vi "Configure Control Mode.vi"(0 "VISA resource name":refnum<visa-resource-name>, 1 "Power Up Enable (F: Off)":bool, 5 "Loop (1:Loop 1)":u16(ring)=1 items=["Loop 1"=1, "Loop 2"=2], 7 "Mode (1:Manual PID)":u16(ring)=1 items=["Manual PID"=1, "Zone"=2, "Open Loop"=3, "AutoTune PID"=4, "AutoTune PI"=5, "AutoTune P"=6], 9 "Control Input (0:A)":u16(ring) items=["A", "B"], 11 "error in (no error)":errorcluster, 12 "Setpoint Units (1:Kelvin)":u16(ring)=1 items=["Kelvin"=1, "Celsius"=2, "Sensor Units"=3], 13 "Heater Output Display (1:Current)":u16(ring)=1 items=["Current"=1, "Power"=2]) -> (4 "VISA resource name out":refnum<visa-resource-name>, 15 "error out":errorcluster)   [LabVIEW 2019, in "Lake Shore 325.lvlib"]
doc: "This VI Specifies the control mode and control loop parameters for the selected loop. The Model 325 has two control modes, Closed Loop and Open Loop. During closed loop control operation the Control Input, Setpoint, Heater Range, PID, and Manual Heater Power (MHP) output parameters are active. Open loop control mode allows the user to directly set the heater output for Loop 1, control output for Loop 2 with the MHP Output parameter.\n\nLoop parameters configured are Input, Setpoint Units, Powerup Enable, and heater output display mode."
uses:
  Lake Shore 325.lvlib
  Instance           2 30Saved   Configure Control Mode .vi
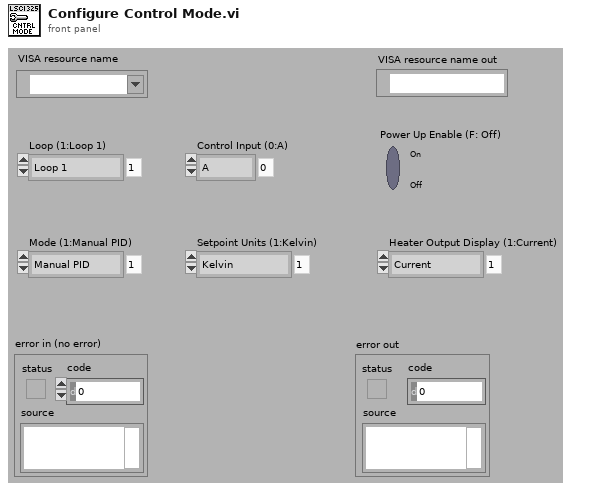
[diagram p1: front panel]
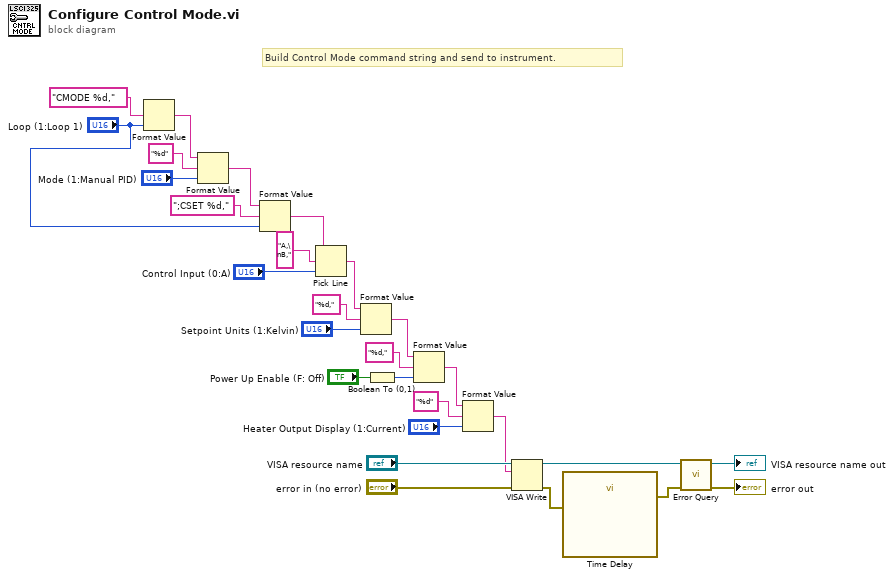
[diagram p0: block diagram]
diagram:
  # "Build Control Mode command string and send to instrument."
  n1 = Format Value(format string="CMODE %d,", value (0)="Loop (1:Loop 1)") -> (output string=w23:string)  [unwired: 1 in]
  n2 = Format Value(string ("")=w23, format string="%d", value (0)="Mode (1:Manual PID)") -> (output string=w18:string)
  n3 = Format Value(string ("")=w18, format string=";CSET %d,", value (0)="Loop (1:Loop 1)") -> (output string=w5:string)
  n4 = Pick Line(string ("")=w5, multi-line string="A,\nB,", line index="Control Input (0:A)") -> (output string=w4:string)
  n5 = Format Value(string ("")=w4, format string="%d,", value (0)="Setpoint Units (1:Kelvin)") -> (output string=w13:string)
  n6 = Boolean To (0,1)(Boolean="Power Up Enable (F: Off)") -> (0, 1=w12:i16)
  n7 = Format Value(string ("")=w13, format string="%d,", value (0)=w12) -> (output string=w9:string)
  n8 = Format Value(string ("")=w9, format string="%d", value (0)="Heater Output Display (1:Current)") -> (output string=w7:string)
  n9 = VISA Write(VISA resource name="VISA resource name", write buffer=w7, error in (no error)="error in (no error)") -> (VISA resource name out=w22:refnum<visa-resource-name>, error out=w2:errorcluster)  [unwired: 1 out]
  n10 = call "Time Delay"("error in (no error)"=w2) -> ("error out"=w1:errorcluster)  [unwired: 10 in]
  n11 = call "Error Query.vi"("error in (no error)"=w1, "VISA resource name"=w22) -> ("error out"=→"error out":errorcluster, "VISA resource name out"=→"VISA resource name out":refnum<visa-resource-name>)  [unwired: 7 in, 1 out]
